vi "New.vi"(6 "Delimiters":cluster{"Close":string, "Open":string}={"Close"="}}", "Open"="{{"}, 8 "Error In":errorcluster, 11 "Key":string) -> (0 "Error Out":errorcluster, 3 "Unescaped Variable":refnum<class "UnescapedVariable.lvclass">)   [LabVIEW 2018, in "Toolkit.lvlib" / "Tokens.lvlib" / "UnescapedVariable.lvclass"]
uses:
  UnescapedVariable.lvclass
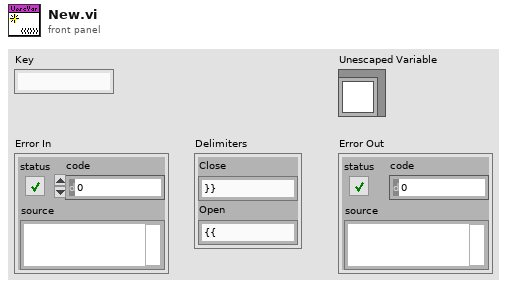
[diagram p1: front panel]
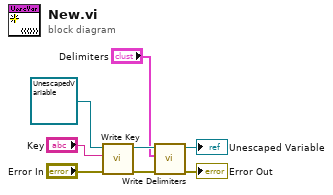
[diagram p0: block diagram]
diagram:
  n1 = call-dynamic "Write Key.vi"("Error In"="Error In", "Key"="Key", "Keyable In"=refnum<class "UnescapedVariable.lvclass"> refnum ("Mustache.lvlib:Tokens.lvlib:UnescapedVariable.lvclass")) -> ("Error Out"=w3:errorcluster, "Keyable Out"=w5:refnum<class "UnescapedVariable.lvclass">)  [unwired: 7 in]
  n2 = call-dynamic "Write Delimiters.vi"("Error In"=w3, "Delimiters"="Delimiters", "Token In"=w5) -> ("Error Out"=→"Error Out":errorcluster, "Token Out"=→"Unescaped Variable":refnum<class "UnescapedVariable.lvclass">)  [unwired: 7 in]
